vi "Reset Device.vi"(11 "Device Name":string="Basys2") -> (0 "Error Out":errorcluster)   [LabVIEW 2011, in "LVH-Adept.lvlib"]
uses:
  <vilib>/LabVIEW Hacker/Adept/LVH-Adept.lvlib
  <vilib>/LabVIEW Hacker/Adept/Private/DMGR/DMGR.lvlib
  <vilib>/LabVIEW Hacker/Adept/Private/DJTG/DJTG.lvlib
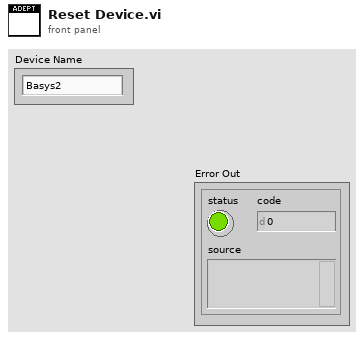
[diagram p1: front panel]
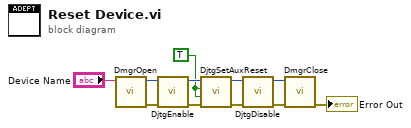
[diagram p0: block diagram]
diagram:
  w1 = TRUE ("Reset Pin Value")
  n1 = call <vilib>:"DmgrOpen.vi"("Device Name"="Device Name") -> ("Error Out"=w3:errorcluster, "Device Handle"=w2:u32)  [unwired: 9 in]
  n2 = call <vilib>:"DjtgEnable.vi"("Error In"=w3, "Device Number"=w2) -> ("Error Out"=w5:errorcluster, "Device Number"=w6:u32)  [unwired: 8 in]
  n3 = call <vilib>:"DjtgSetAuxReset.vi"("Error In"=w5, "Reset Pin Enable"=w1, "Reset Pin Value"=w1, "Device Number"=w6) -> ("Error Out"=w4:errorcluster, "Device Number"=w7:u32)  [unwired: 6 in]
  n4 = call <vilib>:"DjtgDisable.vi"("Error In"=w4, "Device Number"=w7) -> ("Error Out"=w9:errorcluster, "Device Number"=w8:u32)  [unwired: 8 in]
  n5 = call <vilib>:"DmgrClose.vi"("Error In"=w9, "hif"=w8) -> ("Error Out"=→"Error Out":errorcluster)  [unwired: 9 in]
